vi "EnterSerial Number.vi"() -> (0 "Pass/Fail":bool, 1 "ISN":string)   [LabVIEW 2014]
uses:
  <vilib>/event_ctls.llb/eventvkey.ctl
panel:
  in  "ScanISN":T1
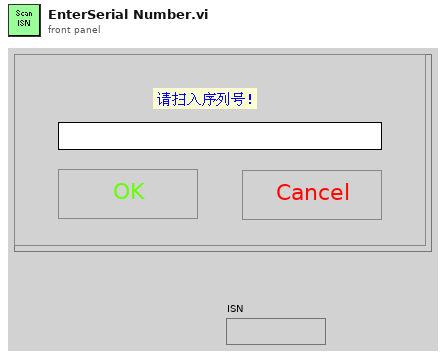
[diagram p1: front panel]
types:
  T1 = cluster{"Pass":bool, "Cancel":bool, "ISN":string}
  T2 = typedef "eventvkey.ctl" = enum16{"ASCII", "Enter", "Return", "Shift", "Ctrl", "Alt", "Cmd", "Opt", "Caps", "NumLock", "Clear", "Break", "Up", "Down", "Left", "Right", "Insert", "Delete", "Home", "End", "PageUp", "PageDown", "Escape", "Help", "Pause", "ScrollLock", "F1", "F2", "F3", "F4", "F5", "F6", "F7", "F8", "F9", "F10", "F11", "F12", "F13", "F14", "F15", "F16", "F17", "F18", "F19", "F20", "F21", "F22", "F23", "F24", "Play", "VolumeUp", "VolumeDown", "Mute", "Two Byte Char"}
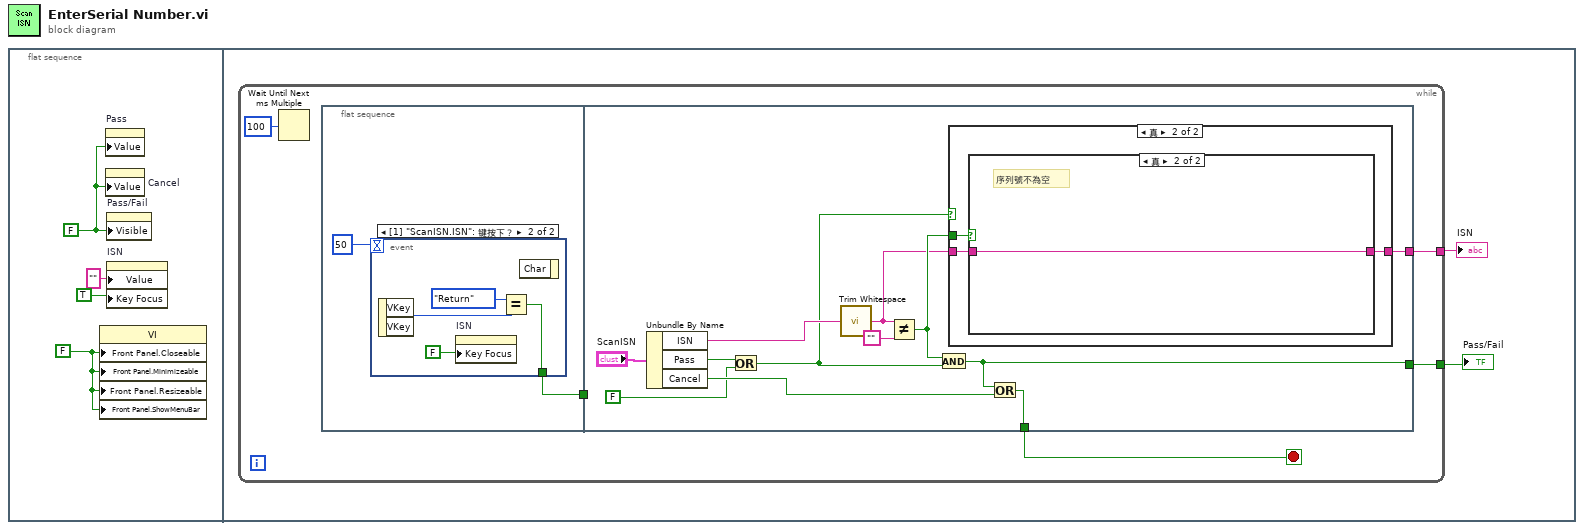
[diagram p0: block diagram]
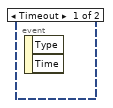
[diagram p2: hidden frame]
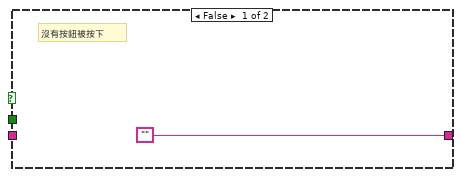
[diagram p3: hidden frame]
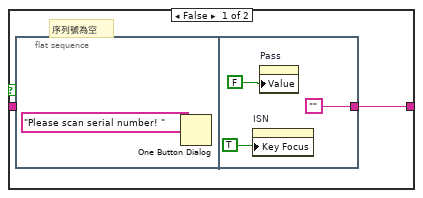
[diagram p4: hidden frame]
diagram:
  n1 = flat-sequence {
    frame #0 {
      w1 = FALSE ("Front Panel Window:Closeable")
      w4 = FALSE ("Visible")
      n2 = property class="VI"("Front Panel.Closeable"=w1, "Front Panel.Minimizeable"=w1, "Front Panel.Resizeable"=w1, "Front Panel.ShowMenuBar"=w1) -> ()  [unwired: 2 in, 2 out]
      n3 = property on="Pass" class="Bool (严格)"("Value"=w4) -> ()  [unwired: 2 in, 2 out]
      n4 = property on="Cancel" class="Bool (严格)"("Value"=w4) -> ()  [unwired: 2 in, 2 out]
      n5 = property on="Pass/Fail" class="Bool (严格)"("Visible"=w4) -> ()  [unwired: 2 in, 2 out]
      n6 = property on="ISN" class="Str"("Value"="", "Key Focus"=TRUE) -> ()  [unwired: 2 in, 2 out]
    }
    frame #1 {
      n7 = while {
        tunnel: [w10] -> w6
        tunnel: [w9] -> w5
        stop <- w8 stop-if-true
        n8 = Wait Until Next ms Multiple(millisecond multiple=i64 100 ("Period")) -> ()  [unwired: 1 out]
        n9 = flat-sequence {
          tunnel: [w12] -> w11
          tunnel: [w26] -> w10
          tunnel: [w24] -> w9
          tunnel: w11 -> [_]
          tunnel: [w21] -> w8
          frame #0 {
            n10 = event shown="[1] \"ScanISN.ISN\": 键按下？" {
              selector: _ -> [_ _]
              dyn-events: _ -> [_ _]
              timeout: 50 -> [_ _]
              tunnel: [_ w14] -> w12
              event Timeout {
                n11 = event-data() -> ()  [unwired: 3 out]
              }
              event "ScanISN.ISN": Key Down? {
                n12 = event-data() -> ("VKey"=w17:T2)  [unwired: 2 out]
                n13 = property on="ISN" class="Str"("Key Focus"=FALSE) -> ()  [unwired: 2 in, 2 out]
                n14 = Equal?(x=eventvkey."Return", y=w17) -> (x = y?=w14:bool)
                n15 = event-data() -> ()  [unwired: 1 in, 2 out]
              }
            }
          }
          frame #1 {
            n16 = Unbundle By Name("ScanISN") -> ("ISN"=w23:string, "Pass"=w20:bool, "Cancel"=w28:bool)
            n17 = Or(x=w20, y=FALSE) -> (x .or. y?=w22:bool)
            n18 = call <vilib>:"Trim Whitespace.vi"("string"=w23) -> ("trimmed string"=w19:string)  [unwired: 1 in]
            n19 = Not Equal?(x=w19, y="") -> (x != y?=w25:bool)
            n20 = And(x=w25, y=w22) -> (x .and. y?=w26:bool)
            n21 = case shown="真" w22 {
              tunnel: w25 -> [_ w33]
              tunnel: ["" w32] -> w24
              tunnel: w19 -> [_ w31]
              frame False {
                # "沒有按鈕被按下"
              }
              frame True {
                n22 = case shown="真" w33 {
                  tunnel: [w34 w39] -> w32
                  tunnel: w31 -> [_ w39]
                  frame False {
                    # "序列號為空"
                    n23 = flat-sequence {
                      tunnel: [""] -> w34
                      frame #0 {
                        n24 = One Button Dialog(message="Please scan serial number! ") -> ()  [unwired: 2 out]
                      }
                      frame #1 {
                        n25 = property on="ISN" class="Str"("Key Focus"=TRUE) -> ()  [unwired: 2 in, 2 out]
                        n26 = property on="Pass" class="Bool (严格)"("Value"=FALSE) -> ()  [unwired: 2 in, 2 out]
                      }
                    }
                  }
                  frame True {
                    # "序列號不為空"
                  }
                }
              }
            }
            n27 = Or(x=w26, y=w28) -> (x .or. y?=w21:bool)
          }
        }
      }
      "Pass/Fail" <- w6
      "ISN" <- w5
    }
  }
